vi "Read Display Format Precision.vi"(8 "error in (no error)":errorcluster, 11 "Digital.lvclass in":refnum<class "Digital.lvclass">) -> (0 "error out":errorcluster, 2 "Precision":u8, 3 "Digital.lvclass out":refnum<class "Digital.lvclass">)   [LabVIEW 2015, in "Digital.lvclass"]
uses:
  Digital.lvclass
  Digital.lvclass/Digital.ctl
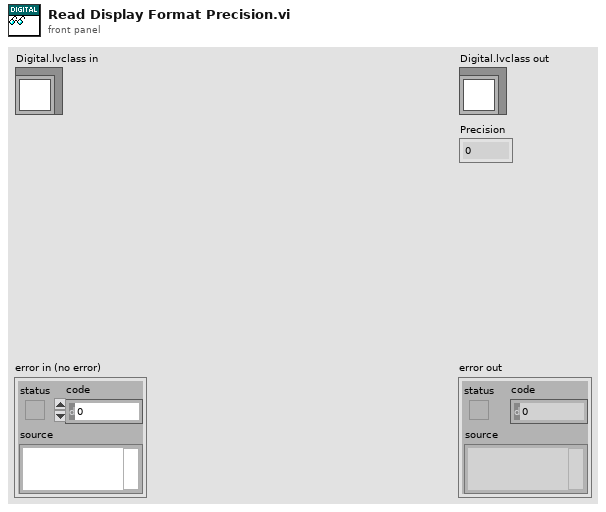
[diagram p1: front panel]
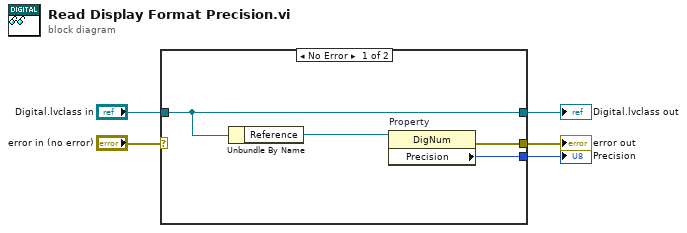
[diagram p0: block diagram]
diagram:
  n1 = case shown="No Error" "error in (no error)" {
    selector: "error in (no error)" -> [_ w11]
    tunnel: [w8 w11] -> w4
    tunnel: [w7 w10] -> w2
    tunnel: "Digital.lvclass in" -> [w7 w10]
    tunnel: [w9 _] -> w1
    frame No Error {
      n2 = Unbundle By Name(w7) -> ("Reference"=w6:refnum<vi>)
      n3 = property on="Property" class="DigNum"(reference=w6) -> (error out=w8:errorcluster, "Precision"=w9:u8)  [unwired: 1 in, 1 out]
    }
    frame Error {
    }
  }
  "error out" <- w4
  "Digital.lvclass out" <- w2
  "Precision" <- w1
